vi "Zoom Attribute.vi"() -> ()   [LabVIEW 2023]
doc: "Illustrates how to use the Zoom Factor property with a 2D Picture. The origin property is also used, and it allows you to programmatically scroll through a picture by referencing the coordinates of the top-left corner of the picture in the picture control."
panel:
  in  "New Origin":cluster{"Horizontal":i16, "Vertical":i16}
  in  "Zoom Factor":sgl(slide)=100.0 min=25 max=200 step=5 scale=25.0..200.0
  in  "Stop":bool
  out "Picture":picture
  # "Overview: Demonstrates how to use the Zoom Factor property to zoom an image in a 2D Picture.\nInstructions:\n1. Run the VI.\n2. Change the Zoom Factor and New Origin controls to manipulate the appearance of the image in the Picture indicator.\n3. Click Stop to stop the VI."
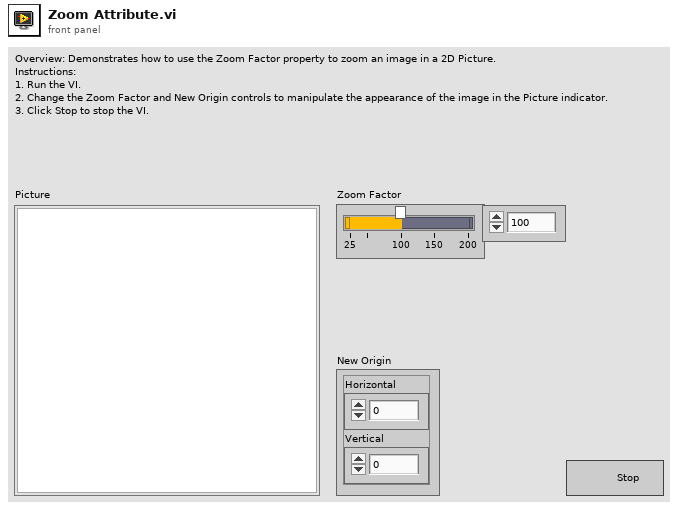
[diagram p1: front panel]
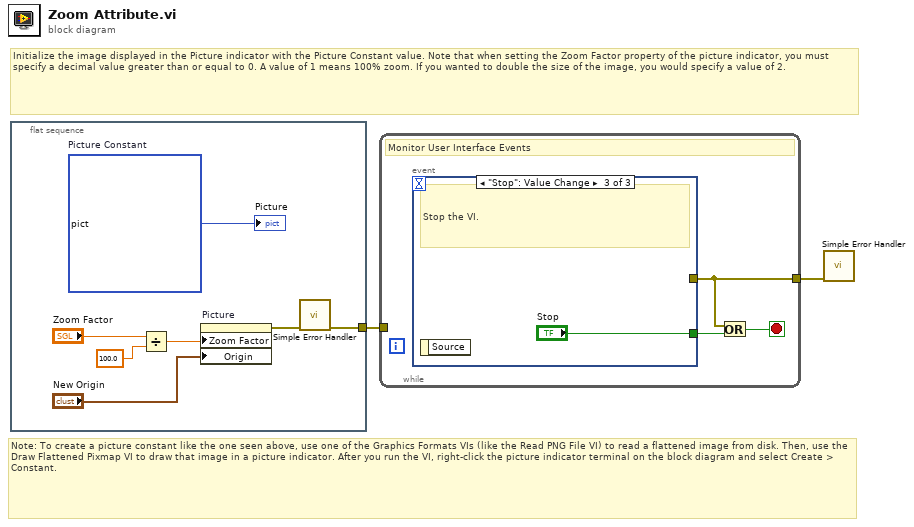
[diagram p0: block diagram]
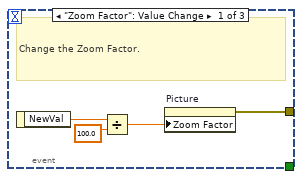
[diagram p2: hidden frame]
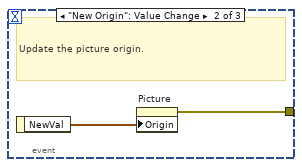
[diagram p3: hidden frame]
diagram:
  # "Note: To create a picture constant like the one seen above, use one of the Graphics Formats VIs (like the Read PNG File VI) to read a flattened image from disk. Then, use the Draw Flattened Pixmap VI to draw that image in a picture indicator. After you run the VI, right-click the picture indicator terminal on the block diagram and select Create > Constant."
  # "Initialize the image displayed in the Picture indicator with the Picture Constant value. Note that when setting the Zoom Factor property of the picture indicator, you must specify a decimal value greater than or equal to 0. A value of 1 means 100% zoom. If you wanted to double the size of the image, you would specify a value of 2."
  n1 = flat-sequence {
    tunnel: [w5] -> w1
    frame #0 {
      w3 = picture bytes[47262]  # Picture Constant
      n2 = Divide(x="Zoom Factor", y=sgl 100.0) -> (x/y=w7:sgl)
      n3 = property on="Picture" class="Picture"("Zoom Factor"=w7, "Origin"="New Origin") -> (error out=w6:errorcluster)  [unwired: 2 in, 1 out]
      n4 = call <vilib>:"Simple Error Handler.vi"("error in (no error)"=w6) -> ("error out"=w5:errorcluster)  [unwired: 4 in, 4 out]
      "Picture" <- w3
    }
  }
  n5 = while {
    tunnel: w1 -> [_]
    tunnel: [w10] -> w2
    stop <- w11 stop-if-true
    # "Monitor User Interface Events"
    n6 = event shown="[2] \"Stop\": Value Change" {
      selector: _ -> [_ _ _]
      dyn-events: _ -> [_ _ _]
      timeout: _ -> [_ _ _]
      tunnel: [_ _ "Stop"] -> w12
      tunnel: [w13 w18 _] -> w10
      event "Zoom Factor": Value Change {
        # "Change the Zoom Factor."
        n7 = event-data() -> ("NewVal"=w14:sgl)  [unwired: 1 in]
        n8 = Divide(x=w14, y=sgl 100.0) -> (x/y=w15:sgl)
        n9 = property on="Picture" class="Picture"("Zoom Factor"=w15) -> (error out=w13:errorcluster)  [unwired: 2 in, 1 out]
      }
      event "New Origin": Value Change {
        # "Update the picture origin."
        n10 = event-data() -> ("NewVal"=w17:cluster{"Horizontal":i16, "Vertical":i16})  [unwired: 1 in]
        n11 = property on="Picture" class="Pict"("Origin"=w17) -> (error out=w18:errorcluster)  [unwired: 2 in, 1 out]
      }
      event "Stop": Value Change {
        # "Stop the VI."
        n12 = event-data() -> ()  [unwired: 1 in, 1 out]
      }
    }
    n13 = Or(x=w10, y=w12) -> (x .or. y?=w11:bool)
  }
  n14 = call <vilib>:"Simple Error Handler.vi"("error in (no error)"=w2) -> ()  [unwired: 4 in, 5 out]
